vi "REPORT_select_path_for_csv_report.vi"(8 "error_in":errorcluster caption="error out", 11 "report_title":string) -> (0 "error_out":errorcluster, 2 "Cancelled?":bool caption="cancelled", 3 "path_to_report":path)   [LabVIEW 2019]
uses:
  _misc/AULocalize/SubVIs/Get Localized Phrase Compact Interface 0D.vi
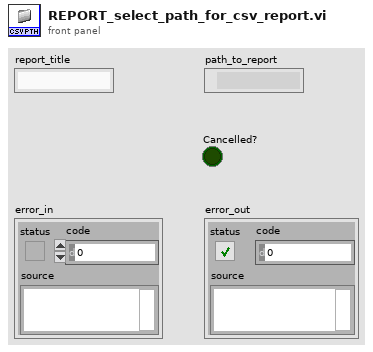
[diagram p1: front panel]
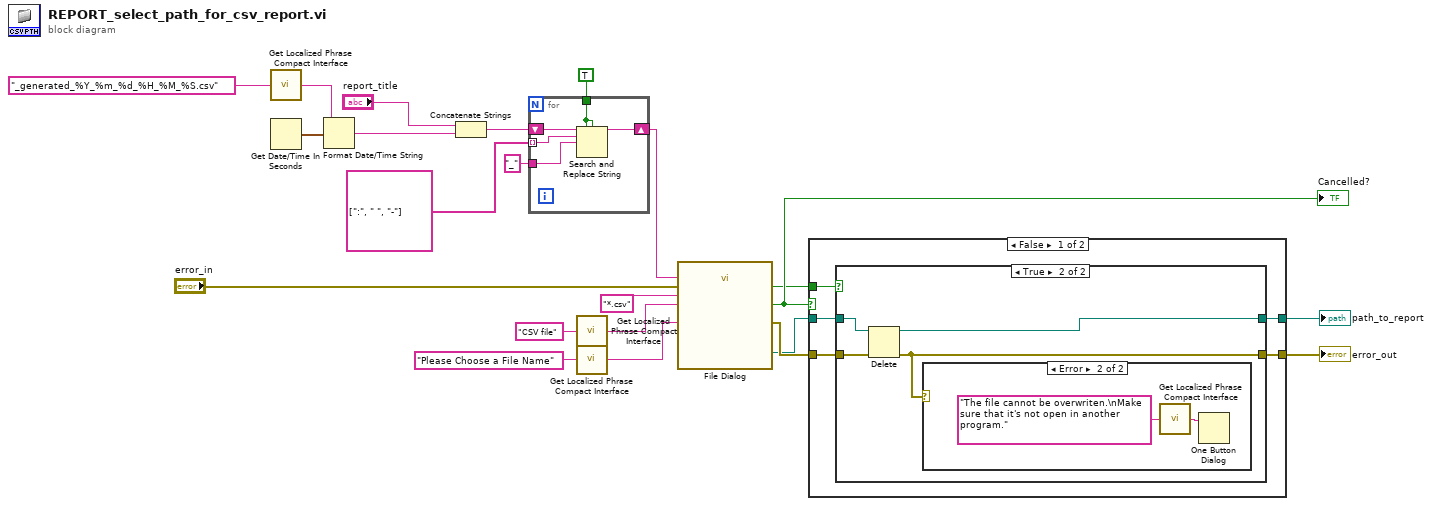
[diagram p0: block diagram]
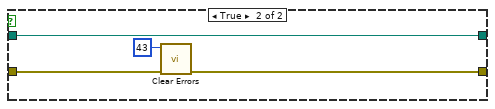
[diagram p4: hidden frame]
diagram:
  n1 = call-poly "Get Localized Phrase Compact Interface.vi"("Key"="_generated_%Y_%m_%d_%H_%M_%S.csv" ("time format string (%c)")) -> ("Translated Phrase"=w1:string)
  n2 = Get Date/Time In Seconds() -> (seconds since 1Jan1904=w14:timestamp)
  n3 = Format Date/Time String(time format string (%c)=w1, seconds (now)=w14) -> (date/time string=w13:string)  [unwired: 1 in]
  n4 = Concatenate Strings("report_title", w13) -> (w8:string)
  n5 = for {
    tunnel: TRUE ("replace all? (F)") -> [w26]
    shift-right: [w25] -> w6
    shift-left: w8 -> [w27]
    tunnel: string[] [":", " ", "-"] -> [w24] mode=indexing
    tunnel: "_" -> [w23]
    n6 = Search and Replace String(replace all?=w26, case sensitive?=w26, input string=w27, search string=w24, replace string=w23) -> (result string=w25:string)  [unwired: 3 in, 3 out]
  }
  n7 = call-poly "Get Localized Phrase Compact Interface.vi"("Key"="CSV file" ("pattern label")) -> ("Translated Phrase"=w3:string)
  n8 = call-poly "Get Localized Phrase Compact Interface.vi"("Key"="Please Choose a File Name" ("prompt")) -> ("Translated Phrase"=w2:string)
  n9 = call "File Dialog"("prompt"=w2, "default name"=w6, "error in"="error_in", "pattern (all files)"="*.csv", "pattern label"=w3) -> ("selected path"=w16:path, "exists"=w18:bool, "cancelled"=w19:bool, "error out"=w17:errorcluster)  [unwired: 2 in, 5 out]
  "Cancelled?" <- w19
  n10 = case shown="False" w19 {
    tunnel: w18 -> [w32 _]
    tunnel: w17 -> [w31 w43]
    tunnel: w16 -> [w30 w44]
    tunnel: [w29 w42] -> w10
    tunnel: [w28 w44] -> w11
    frame False {
      n11 = case shown="True" w32 {
        tunnel: w31 -> [w33 w38]
        tunnel: w30 -> [w34 w37]
        tunnel: [w33 w35] -> w29
        tunnel: [w34 w36] -> w28
        frame False {
        }
        frame True {
          n12 = Delete(path (use dialog)=w37, error in=w38) -> (deleted path=w36:path, error out=w35:errorcluster)  [unwired: 4 out]
          n13 = case shown="Error" w35 {
            frame No Error {
            }
            frame Error {
              n14 = call-poly "Get Localized Phrase Compact Interface.vi"("Key"="The file cannot be overwriten.\nMake sure that it's not open in another program." ("prompt")) -> ("Translated Phrase"=w39:string)
              n15 = One Button Dialog(message=w39) -> ()  [unwired: 2 out]
            }
          }
        }
      }
    }
    frame True {
      n16 = call <vilib>:"Clear Errors.vi"("error in (no error)"=w43, "specific error code to clear (0: all)"=43) -> ("error out"=w42:errorcluster)  [unwired: 4 in, 1 out]
    }
  }
  "path_to_report" <- w11
  "error_out" <- w10
